vi "RobotSimulatorAvancedAtt.vi"() -> ()   [LabVIEW 2020]
uses:
  a11d5919-bfa0-408a-bf71-221d1caa9c76.vi
  <vilib>/Utility/inputDevices.llb/joystickAcquire.vi
  <vilib>/Utility/inputDevices.llb/closeJoystick.vi
panel:
  out "Garra Inclinação":u8(slide) scale=0.0..100.0
  out "Ativ.":bool
  out "?":dbl(knob) scale=-100.0..100.0 scale format="%#.1f"
  out "Trás Esq.":bool
  out "Frente Dir.":bool
  out "Trás Dir.":bool
  out "Frente Esq.":bool
  out "joystick info":T1(array[cluster])
  out "direction info":T2
  out "button info":T3
  out "axis info":T4
  # "Velocidade"
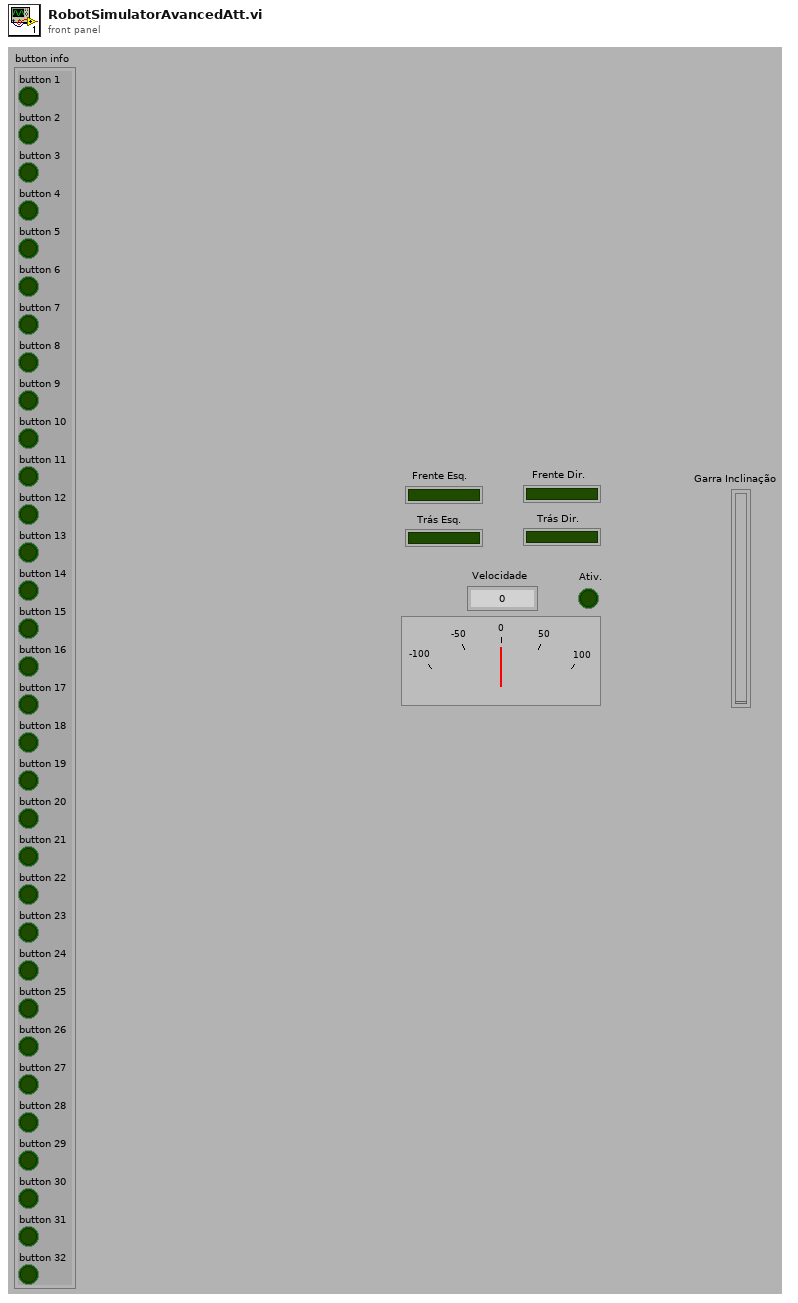
[diagram p1: front panel]
types:
  T1 = cluster{"axes total":u32, "buttons total":u32, "pov total":u32, "device name":string}[]
  T2 = cluster{"pov 1":i32, "pov 2":i32, "pov 3":i32, "pov 4":i32}
  T3 = cluster{"button 1":bool, "button 2":bool, "button 3":bool, "button 4":bool, "button 5":bool, "button 6":bool, "button 7":bool, "button 8":bool, "button 9":bool, "button 10":bool, "button 11":bool, "button 12":bool, "button 13":bool, "button 14":bool, "button 15":bool, "button 16":bool, "button 17":bool, "button 18":bool, "button 19":bool, "button 20":bool, "button 21":bool, "button 22":bool, "button 23":bool, "button 24":bool, "button 25":bool, "button 26":bool, "button 27":bool, "button 28":bool, "button 29":bool, "button 30":bool, "button 31":bool, "button 32":bool}
  T4 = cluster{"X axis":i32, "Y axis":i32, "Z axis":i32, "X axis rotation":i32, "Y axis rotation":i32, "Z axis rotation":i32, "U axis":i32, "V axis":i32}
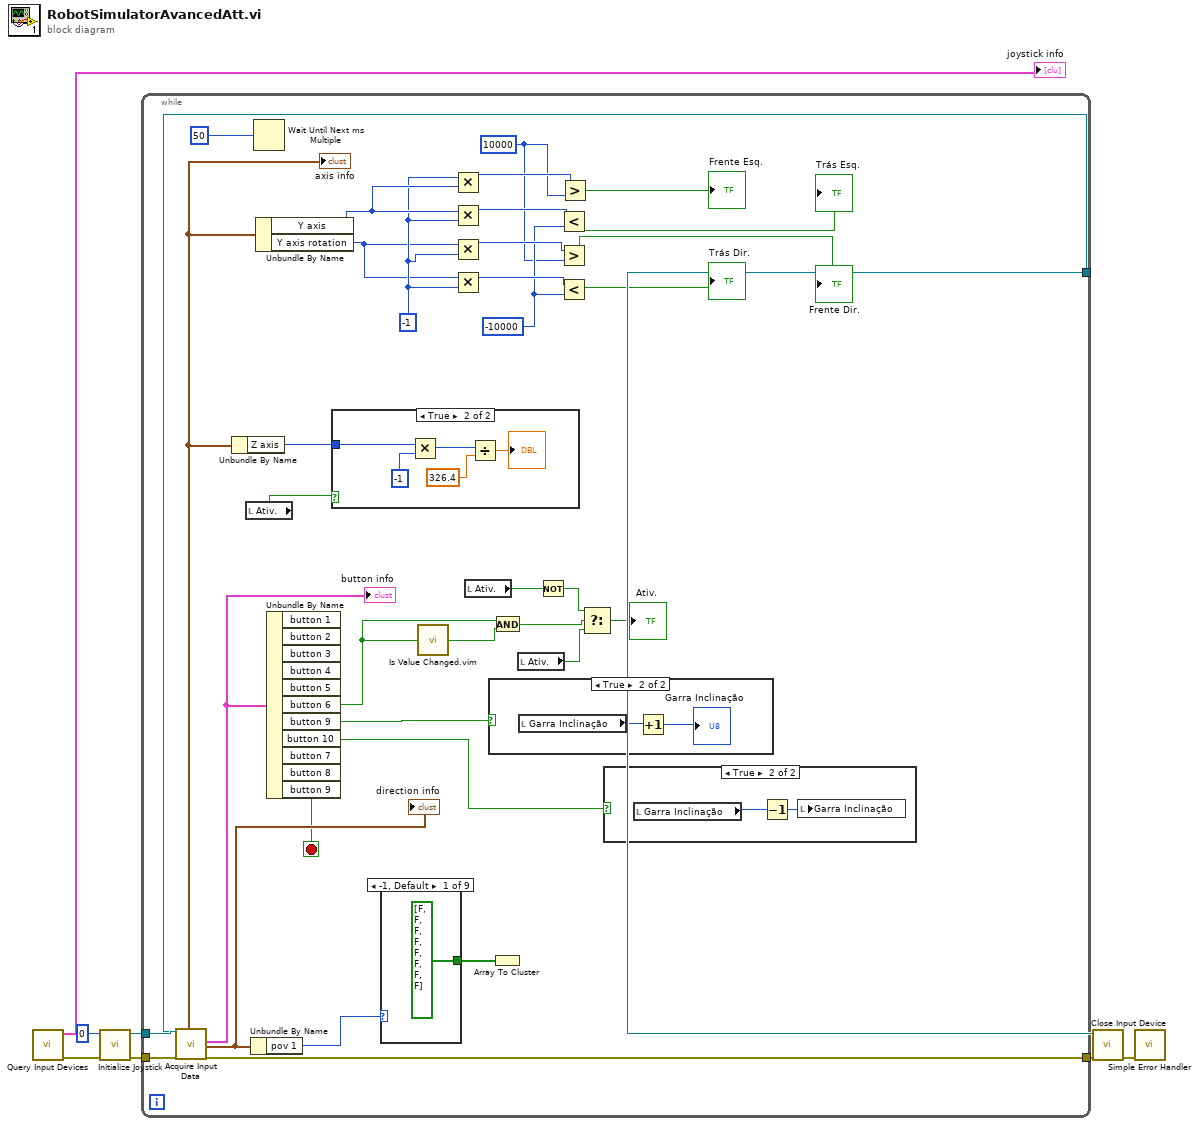
[diagram p0: block diagram]
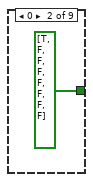
[diagram p5: hidden frame]
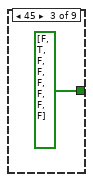
[diagram p6: hidden frame]
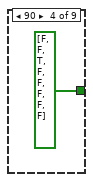
[diagram p7: hidden frame]
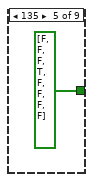
[diagram p8: hidden frame]
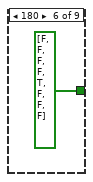
[diagram p9: hidden frame]
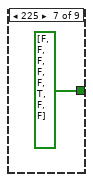
[diagram p10: hidden frame]
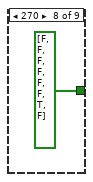
[diagram p11: hidden frame]
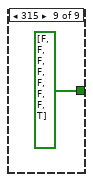
[diagram p12: hidden frame]
diagram:
  n1 = call <vilib>:"Query Input Devices.vi"() -> ("error out"=w2:errorcluster, "joystick info"=→"joystick info":T1)  [unwired: 1 in, 9 out]
  n2 = call <vilib>:"Initialize Joystick.vi"("error in (no error)"=w2, "device index"=0) -> ("error out"=w6:errorcluster, "device ID"=w7:refnum<k1>)  [unwired: 8 out]
  n3 = while {
    tunnel: w7 -> [w43]
    tunnel: w6 -> [w42]
    tunnel: [w41] -> w5
    tunnel: [w36] -> w4
    stop <- w35 stop-if-true
    w21 = 10000
    w22 = -10000
    w31 = -1
    n4 = call-poly <vilib>:"Acquire Input Data.vi"("device ID"=w43, "error in (no error)"=w42) -> ("device ID"=w41:refnum<k1>, "axis info"=w33:T4, "button info"=w40:T3, "direction info"=w39:T2, "error out"=w36:errorcluster)  [unwired: 13 out]
    "axis info" <- w33
    "button info" <- w40
    "direction info" <- w39
    n5 = Unbundle By Name(w33) -> ("Z axis"=w19:i32)
    n6 = local read "Ativ."() -> (w18:bool)
    n7 = Unbundle By Name(w39) -> ("pov 1"=w38:i32)
    n8 = Wait Until Next ms Multiple(millisecond multiple=u32 50) -> ()  [unwired: 1 out]
    n9 = Unbundle By Name(w33) -> ("Y axis"=w32:i32, "Y axis rotation"=w30:i32)
    n10 = Unbundle By Name(w40) -> ("button 6"=w16:bool, "button 9"=w10:bool, "button 10"=w9:bool, "button 7"=w35:bool)  [unwired: 7 out]
    n11 = case shown="True" w18 {
      tunnel: w19 -> [_ w48]
      frame False {
      }
      frame True {
        n12 = Multiply(x=w48, y=-1) -> (x*y=w52:i32)
        n13 = Divide(x=w52, y=326.4) -> (x/y=→"?":dbl)
      }
    }
    n14 = case shown="-1, Default" w38 {
      tunnel: [bool[] [FALSE, FALSE, FALSE, FALSE, FALSE, FALSE, FALSE, FALSE] ("Array") bool[] [TRUE, FALSE, FALSE, FALSE, FALSE, FALSE, FALSE, FALSE] ("Array") bool[] [FALSE, TRUE, FALSE, FALSE, FALSE, FALSE, FALSE, FALSE] ("Array") bool[] [FALSE, FALSE, TRUE, FALSE, FALSE, FALSE, FALSE, FALSE] ("Array") bool[] [FALSE, FALSE, FALSE, TRUE, FALSE, FALSE, FALSE, FALSE] ("Array") bool[] [FALSE, FALSE, FALSE, FALSE, TRUE, FALSE, FALSE, FALSE] ("Array") bool[] [FALSE, FALSE, FALSE, FALSE, FALSE, TRUE, FALSE, FALSE] ("Array") bool[] [FALSE, FALSE, FALSE, FALSE, FALSE, FALSE, TRUE, FALSE] ("Array") bool[] [FALSE, FALSE, FALSE, FALSE, FALSE, FALSE, FALSE, TRUE] ("Array")] -> w37
      frame -1, Default {
      }
      frame 0 {
      }
      frame 45 {
      }
      frame 90 {
      }
      frame 135 {
      }
      frame 180 {
      }
      frame 225 {
      }
      frame 270 {
      }
      frame 315 {
      }
    }
    n15 = call "Is Value Changed.vim"("value"=w16) -> ("changed or first call?"=w17:bool)
    n16 = Multiply(x=w31, y=w32) -> (x*y=w23:i32)
    n17 = Multiply(x=w32, y=w31) -> (x*y=w26:i32)
    n18 = Multiply(x=w30, y=w31) -> (x*y=w28:i32)
    n19 = Multiply(x=w30, y=w31) -> (x*y=w27:i32)
    n20 = local read "Ativ."() -> (w14:bool)
    n21 = case shown="True" w10 {
      frame False {
      }
      frame True {
        n22 = local read "Garra Inclinação"() -> (w47:u8)
        n23 = Increment(x=w47) -> (x+1=→"Garra Inclinação":u8)
      }
    }
    n24 = Array To Cluster(array=w37) -> ()  [unwired: 1 out]
    n25 = And(x=w16, y=w17) -> (x .and. y?=w15:bool)
    n26 = local read "Ativ."() -> (w12:bool)
    n27 = Not(x=w14) -> (.not. x?=w13:bool)
    n28 = Less?(x=w26, y=w22) -> (x < y?=→"Trás Esq.":bool)
    n29 = Greater?(x=w28, y=w21) -> (0:→"Frente Dir.":bool)
    n30 = Less?(x=w27, y=w22) -> (x < y?=→"Trás Dir.":bool)
    n31 = Greater?(x=w23, y=w21) -> (0:→"Frente Esq.":bool)
    n32 = Select(t=w13, s=w15, f=w12) -> (s? t:f=→"Ativ.":bool)
    n33 = case shown="True" w9 {
      frame False {
      }
      frame True {
        n34 = local read "Garra Inclinação"() -> (w44:u8)
        n35 = Decrement(x=w44) -> (x-1=w45:u8)
        n36 = local write "Garra Inclinação"(w45) -> ()
      }
    }
  }
  n37 = call-poly <vilib>:"Close Input Device.vi"("error in (no error)"=w4, "device ID"=w5) -> ("error out"=w1:errorcluster)  [unwired: 8 out]
  n38 = call <vilib>:"Simple Error Handler.vi"("error in (no error)"=w1) -> ()  [unwired: 1 in, 8 out]
